vi "SubVI_ReadMatS_001.vi"(11 "1-bit pixmap   in":bool[][](array[boolean])) -> (2 "array of inputs":bool[](array[boolean]), 3 "total #iter":i32)   [LabVIEW 2018]
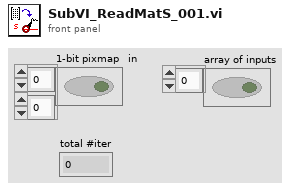
[diagram p1: front panel]
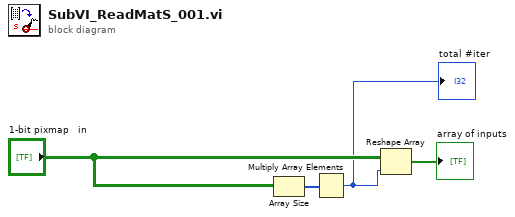
[diagram p0: block diagram]
diagram:
  n1 = Array Size(array="1-bit pixmap   in") -> (size(s)=w1:i32[])
  n2 = Multiply Array Elements(1:w1) -> (0:w3:i32)
  "total #iter" <- w3
  n3 = Reshape Array("1-bit pixmap   in", w3) -> (→"array of inputs":bool[])
